vi "Swerve_Get_ Bot_State.vi"(10 "Mod Ref":string[](array[string]), 11 "refnum name":string) -> (2 "Mod Pos":T1[](array[typedef]) {"Angle"."SIN" format="%13.4f"; "Angle"."COS" format="%13.4f"; "Angle"."VALUE" format="%13.4f"}, 3 "Mod State":T3[](array[typedef]) {"Angle"."SIN" format="%13.4f"; "Angle"."COS" format="%13.4f"; "Angle"."VALUE" format="%13.4f"})   [LabVIEW 2020]
uses:
  <vilib>/Rock Robotics/WPI/ThirdParty/JAS_Junk/TrajLib/TypeDef/SWERVE_DRIVE_MODULE_STATE.ctl
  <vilib>/Rock Robotics/WPI/ThirdParty/JAS_Junk/TrajLib/TypeDef/ROTATION2D.ctl
  <vilib>/Rock Robotics/WPI/ThirdParty/JAS_Junk/TrajLib/TypeDef/SWERVE_DRIVE_MODULE_POSITION.ctl
  <vilib>/Rock Robotics/WPI/Joystick/XBox Buttons Indexer.ctl
  Robot Global Data.vi
  <vilib>/Rock Robotics/WPI/ThirdParty/JAS_Junk/TrajLib/Trajectory_Library.lvlib
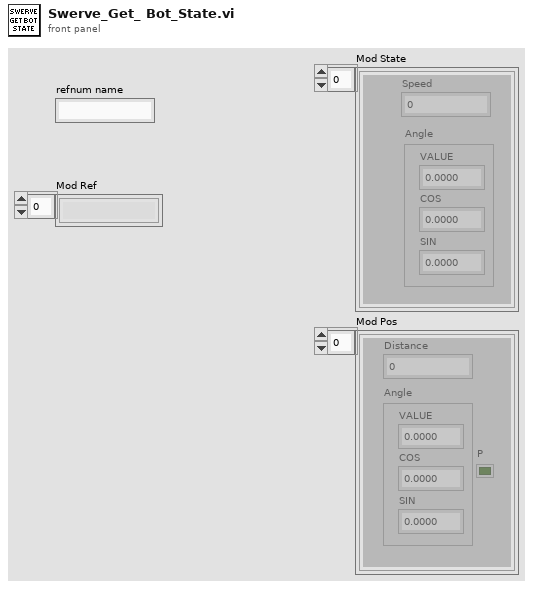
[diagram p1: front panel]
types:
  T1 = typedef "Trajectory_Library.lvlib/SWERVE_DRIVE_MODULE_POSITION.ctl" = cluster{"Distance":dbl, "Angle":T2, "P":bool}
  T2 = typedef "Trajectory_Library.lvlib/ROTATION2D.ctl" = cluster{"VALUE":dbl, "COS":dbl, "SIN":dbl}
  T3 = typedef "Trajectory_Library.lvlib/SWERVE_DRIVE_MODULE_STATE.ctl" = cluster{"Speed":dbl, "Angle":T2}
  T4 = typedef "XBox Buttons Indexer.ctl" = enum16{"A", "B", "X", "Y", "Left Bumper", "Right Bumper", "Back", "Start", "Left Joystick", "Right Joystick"}
  T5 = typedef "WPI_GyroDevRef.ctl" = cluster{"DevStatus":errorcluster, "Analog Channel":T6, "Gain (VoltsPerDegree/Second)":dbl, "Gyro Type":enum16{"Analog", "XRS450"}, "Handle":i32, "SPI Bus":T7, "Device Found":bool, "Sample Rate":dbl, "Calibrate On Open":bool, "Offset":dbl}
  T6 = typedef "FPGA_AIChannel.ctl" = enum8{"AI 0", "AI 1", "AI 2", "AI 3", "AI MXP 0", "AI MXP 1", "AI MXP 2", "AI MXP 3", "Invalid"}
  T7 = typedef "spi_bus.ctl" = enum16{"SPI On-Board, CS0", "SPI On-Board, CS1", "SPI On-Board, CS2", "SPI On-Board, CS3", "SPI MXP", "Invalid"}
  T8 = typedef "Trajectory_Library.lvlib/SWERVE_DRIVE_KINEMATICS.ctl" = cluster{"NumModules":i32, "InverseKinematics":T9, "ForwardKinematics":T9, "Modules":T10[], "PrevCoR":T10, "SavedModuleStates":T3[]}
  T9 = typedef "NI_Matrix.lvlib/RealMatrix.ctl" = dbl[][]
  T10 = typedef "Trajectory_Library.lvlib/TRANSLATION2D.ctl" = cluster{"X":dbl, "Y":dbl}
  T11 = typedef "Trajectory_Library.lvlib/CHASSIS_SPEEDS.ctl" = cluster{"vX":dbl, "vY":dbl, "vOmega":dbl}
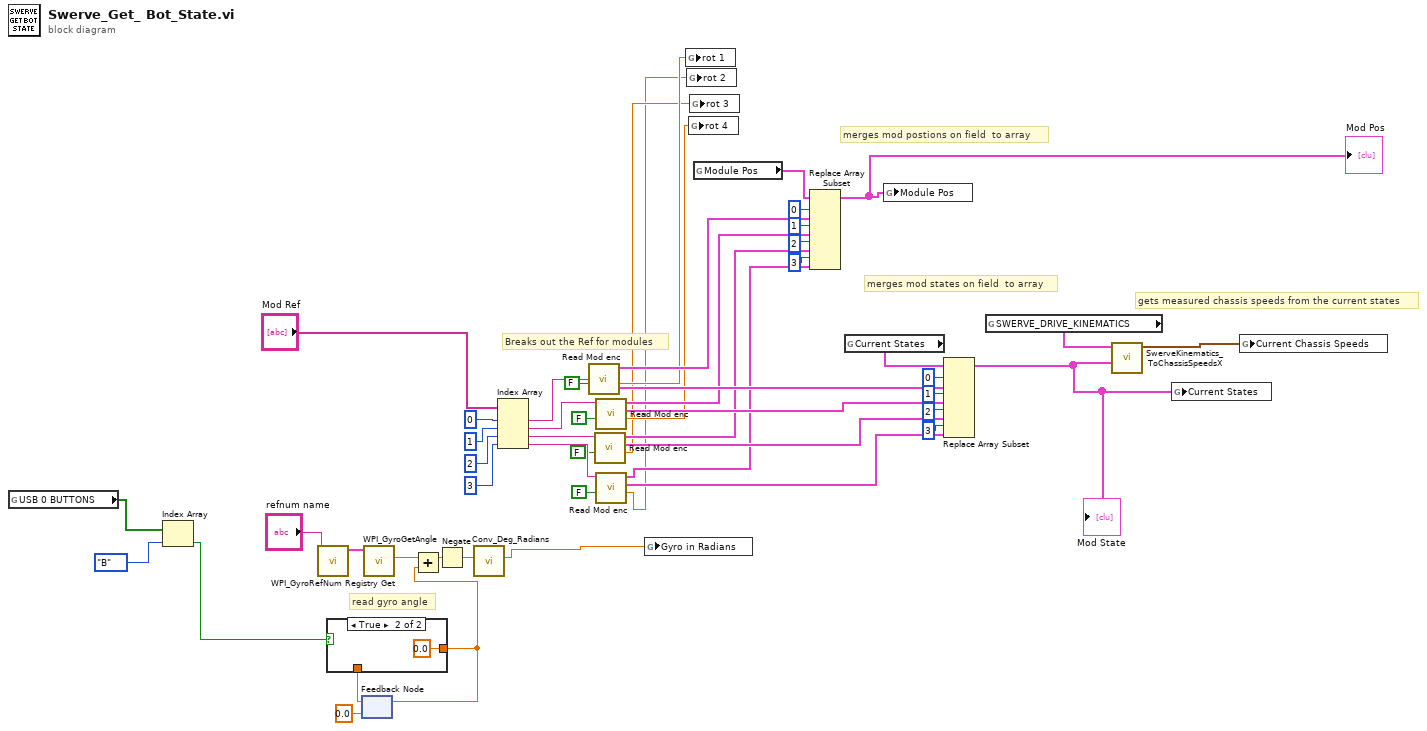
[diagram p0: block diagram]
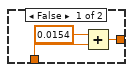
[diagram p2: hidden frame]
diagram:
  # "gets measured chassis speeds from the current states"
  # "merges mod states on field  to array"
  # "merges mod postions on field  to array"
  # "read gyro angle"
  # "Breaks out the Ref for modules"
  n1 = global read "Robot Global Data.vi" "USB 0 BUTTONS"() -> (w3:bool[])
  n2 = Index Array(array=w3, index=XBox_Buttons_Indexer."B" ("XBox Buttons")) -> (element=w1:bool)
  n3 = call <vilib>:"WPI_GyroRefNum Registry Get.vi"("refnum name"="refnum name") -> ("GyroDevRef"=w39:T5)  [unwired: 9 in, 1 out]
  n4 = feedback #1(0.0) -> (w7:dbl)
  n5 = case shown="True" w1 {
    tunnel: w7 -> [w54 _]
    tunnel: [w52 0.0] -> w4
    frame False {
      n6 = Add(x=0.0154, y=w54) -> (x+y=w52:dbl)
    }
    frame True {
    }
  }
  n7 = feedback-in #1(w4) -> ()
  n8 = call <vilib>:"WPI_GyroGetAngle.vi"("GyroDevRef"=w39) -> ("Angle"=w41:dbl)  [unwired: 6 in, 4 out]
  n9 = Add(x=w41, y=w4) -> (x+y=w5:dbl)
  n10 = Negate(x=w5) -> (-x=w40:dbl)
  n11 = call <vilib>:"Conv_Deg_Radians.vi"("Degress"=w40) -> ("Radians"=w12:dbl)  [unwired: 10 in]
  n12 = Index Array(array="Mod Ref", index #1=0 ("index"), index #2=1 ("index"), index #3=2 ("index"), index #4=3 ("index")) -> (element #1=w51:string, element #2=w48:string, element #3=w49:string, element #4=w50:string)
  n13 = call "Read Mod enc.vi"("invert"=FALSE, "Mod Ref"=w51) -> ("rot angle"=w16:dbl, "SWERVE_DRIVE_MODULE_STATE"=w32:T3, "SWERVE_DRIVE_MODULE_POSITION"=w20:T1)  [unwired: 7 in]
  n14 = call "Read Mod enc.vi"("invert"=FALSE, "Mod Ref"=w49) -> ("rot angle"=w14:dbl, "SWERVE_DRIVE_MODULE_STATE"=w34:T3, "SWERVE_DRIVE_MODULE_POSITION"=w18:T1)  [unwired: 7 in]
  n15 = call "Read Mod enc.vi"("invert"=FALSE, "Mod Ref"=w48) -> ("rot angle"=w15:dbl, "SWERVE_DRIVE_MODULE_STATE"=w33:T3, "SWERVE_DRIVE_MODULE_POSITION"=w19:T1)  [unwired: 7 in]
  n16 = call "Read Mod enc.vi"("invert"=FALSE, "Mod Ref"=w50) -> ("rot angle"=w13:dbl, "SWERVE_DRIVE_MODULE_STATE"=w35:T3, "SWERVE_DRIVE_MODULE_POSITION"=w17:T1)  [unwired: 7 in]
  n17 = global write "Robot Global Data.vi" "Gyro in Radians"(w12) -> ()
  n18 = global write "Robot Global Data.vi" "rot 1"(w16) -> ()
  n19 = global write "Robot Global Data.vi" "rot 2"(w13) -> ()
  n20 = global write "Robot Global Data.vi" "rot 4"(w15) -> ()
  n21 = global write "Robot Global Data.vi" "rot 3"(w14) -> ()
  n22 = global read "Robot Global Data.vi" "Module Pos"() -> (w22:T1[])
  n23 = Replace Array Subset(array=w22, new element #1=w20, index #1=0 ("index"), new element #2=w19, index #2=1 ("index"), new element #3=w18, index #3=2 ("index"), new element #4=w17, index #4=3 ("index")) -> (w21:T1[])
  "Mod Pos" <- w21
  n24 = global read "Robot Global Data.vi" "Current States"() -> (w27:T3[])
  n25 = global write "Robot Global Data.vi" "Module Pos"(w21) -> ()
  n26 = Replace Array Subset(array=w27, new element #1=w32, index #1=0 ("index"), new element #2=w33, index #2=1 ("index"), new element #3=w34, index #3=2 ("index"), new element #4=w35, index #4=3 ("index")) -> (w36:T3[])
  "Mod State" <- w36
  n27 = global read "Robot Global Data.vi" "SWERVE_DRIVE_KINEMATICS"() -> (w37:T8)
  n28 = call <vilib>:"SwerveKinematics_ToChassisSpeedsX.vi"("WheelStates"=w36, "in SWERVE_DRIVE_KINEMATICS"=w37) -> ("Chassis Speed"=w38:T11)  [unwired: 9 in]
  n29 = global write "Robot Global Data.vi" "Current States"(w36) -> ()
  n30 = global write "Robot Global Data.vi" "Current Chassis Speeds"(w38) -> ()
